vi "GetStopUE.vi"(8 "Error In":errorcluster) -> (0 "Error Out":errorcluster, 3 "STOP":refnum<user-event>)   [LabVIEW 2017, in "StopUE.lvlib"]
uses:
  StopUE.lvlib
  States_FGV.ctl
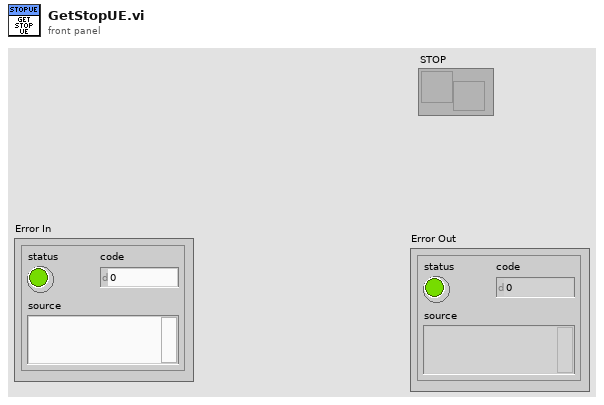
[diagram p1: front panel]
types:
  T1 = typedef "StopUE.lvlib/States_FGV.ctl" = enum16{"Get", "Shutdown", "Initialize"}
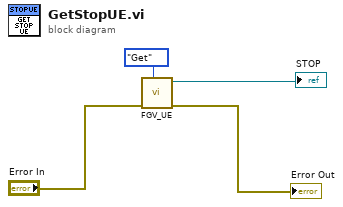
[diagram p0: block diagram]
diagram:
  n1 = call "FGV_UE.vi"("State"=States_FGV."Get", "Error In"="Error In") -> ("Error Out"=→"Error Out":errorcluster, "STOP"=→"STOP":refnum<user-event>)  [unwired: 8 in]
